vi "Periodic Tasks.vi"(8 "error in":errorcluster) -> ()   [LabVIEW 2017]
doc: "This VI runs in parallel to other tasks. It can contain as many user-defined periodic loops as you need. These can carry out PID or other sorts of timed response."
uses:
  <vilib>/Rock Robotics/WPI/Utilities/WPI_GetSetVariantRefNum.vi
  Robot Global Data.vi
  <vilib>/Rock Robotics/Network Tables/NT Write Numeric Array.vi
  <vilib>/Rock Robotics/Network Tables/NT Write Number.vi
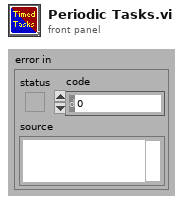
[diagram p1: front panel]
types:
  T1 = typedef "WPI_MotorControlDeviceRef.ctl" = cluster{"DeviceStatus":errorcluster, "Type":T2, "PWM":cluster{"PWM Channel":T3, "DeadBand":T4}, "CAN":cluster{"Device Number":u8, "SetOutput VI Ref":variant, "GetOutput VI Ref":variant, "Enable VI Ref":variant, "Disable VI Ref":variant, "Data":variant}, "Invert":bool, "DIO PWM":cluster{"PWM \"Enable\" Channel":T3, "DIOChannel":T5, "PWM Rate":dbl}}
  T2 = typedef "WPI_MotorControlType.ctl" = enum16{"PWM", "CAN", "DIO PWM"}
  T3 = typedef "FPGA_DIOPWMChannel.ctl" = enum8{"PWM 0", "PWM 1", "PWM 2", "PWM 3", "PWM 4", "PWM 5", "PWM 6", "PWM 7", "PWM 8", "PWM 9", "PWM MXP 0", "PWM MXP 1", "PWM MXP 2", "PWM MXP 3", "PWM MXP 4", "PWM MXP 5", "PWM MXP 6", "PWM MXP 7", "PWM MXP 8", "PWM MXP 9", "Invalid"}
  T4 = typedef "WPI_PWMDeadband.ctl" = cluster{"Name":string, "maxPositivePwm":i32, "minPositivePwm":i32, "centerPwm":i32, "maxNegativePwm":i32, "minNegativePwm":i32, "angularRange":u16}
  T5 = typedef "FPGA_DIOChannel.ctl" = enum8{"DIO 0", "DIO 1", "DIO 2", "DIO 3", "DIO 4", "DIO 5", "DIO 6", "DIO 7", "DIO 8", "DIO 9", "DIO MXP 0", "DIO MXP 1", "DIO MXP 2", "DIO MXP 3", "DIO MXP 4", "DIO MXP 5", "DIO MXP 6", "DIO MXP 7", "DIO MXP 8", "DIO MXP 9", "DIO MXP 10", "DIO MXP 11", "DIO MXP 12", "DIO MXP 13", "DIO MXP 14", "DIO MXP 15", "SPI Port CS1", "SPI Port CS2", "SPI Port CS3", "SPI Port MISO", "SPI Port MOSI", "Invalid"}
  T6 = typedef "WPI_RobotDriveDevRef.ctl" = cluster{"DevStatus":errorcluster, "Motors[]":T1[], "Square Inputs":bool, "Max Output":dbl}
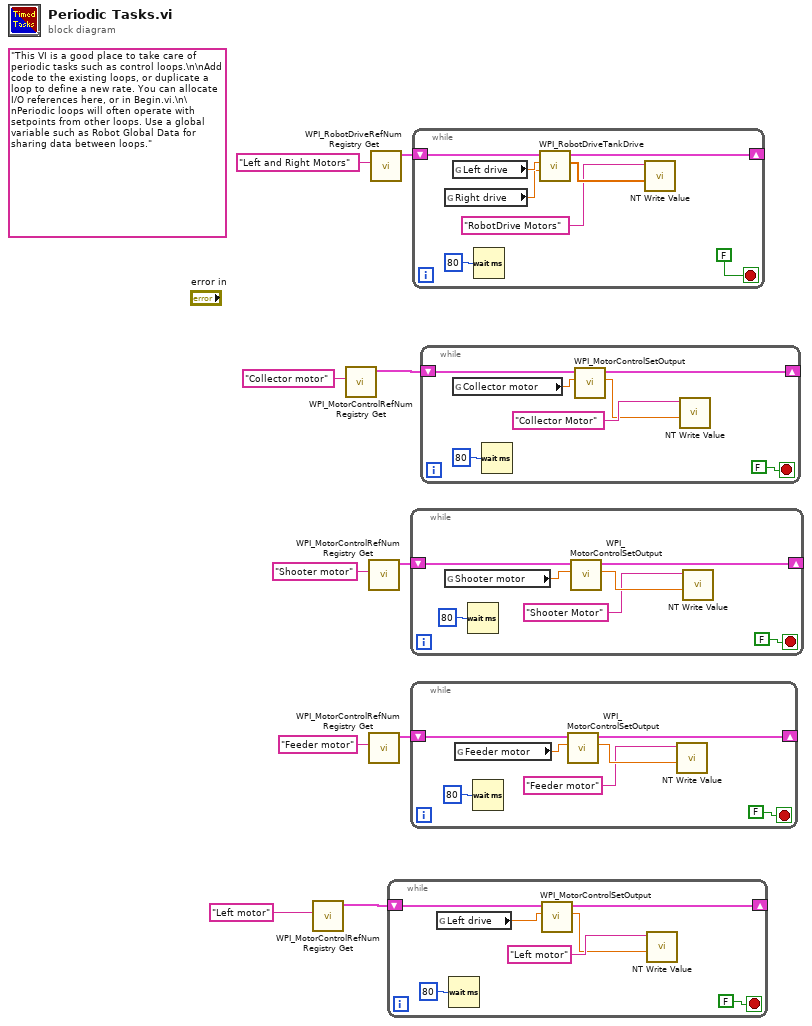
[diagram p0: block diagram]
diagram:
  (unwired) "This VI is a good place to take care of periodic tasks such as control loops.\n\nAdd code to the existing loops, or duplicate a loop to define a new rate. You can allocate I/O references here, or in Begin.vi.\n\nPeriodic loops will often operate with setpoints from other loops. Use a global variable such as Robot Global Data for sharing data between loops."
  n1 = call <vilib>:"WPI_MotorControlRefNum Registry Get.vi"("refnum name"="Left motor") -> ("MotorControlDevRef"=w2:T1)  [unwired: 9 in, 1 out]
  n2 = call <vilib>:"WPI_MotorControlRefNum Registry Get.vi"("refnum name"="Collector motor") -> ("MotorControlDevRef"=w5:T1)  [unwired: 9 in, 1 out]
  n3 = call <vilib>:"WPI_MotorControlRefNum Registry Get.vi"("refnum name"="Shooter motor") -> ("MotorControlDevRef"=w6:T1)  [unwired: 9 in, 1 out]
  n4 = call <vilib>:"WPI_MotorControlRefNum Registry Get.vi"("refnum name"="Feeder motor") -> ("MotorControlDevRef"=w3:T1)  [unwired: 9 in, 1 out]
  n5 = call <vilib>:"WPI_RobotDriveRefNum Registry Get.vi"("refnum name"="Left and Right Motors") -> ("RobotDriveDevRef"=w9:T6)  [unwired: 1 in, 9 out]
  n6 = while {
    shift-right: [w11] -> _
    shift-left: w2 -> [w12]
    stop <- FALSE stop-if-true
    n7 = global read "Robot Global Data.vi" "Left drive"() -> (w13:dbl)
    n8 = Wait (ms)(milliseconds to wait=u32 80) -> ()  [unwired: 1 out]
    n9 = call <vilib>:"WPI_MotorControlSetOutput.vi"("Output"=w13, "MotorControlDevRef"=w12) -> ("Motor Output"=w14:dbl, "MotorControlDevRef"=w11:T1)  [unwired: 7 in, 1 out]
    n10 = call-poly <vilib>:"NT Write Value.vi"("Numeric"=w14, "Name"="Left motor") -> ()  [unwired: 9 in, 1 out]
  }
  n11 = while {
    shift-right: [w20] -> _
    shift-left: w6 -> [w19]
    stop <- FALSE stop-if-true
    n12 = global read "Robot Global Data.vi" "Shooter motor"() -> (w22:dbl)
    n13 = Wait (ms)(milliseconds to wait=u32 80) -> ()  [unwired: 1 out]
    n14 = call <vilib>:"WPI_MotorControlSetOutput.vi"("Output"=w22, "MotorControlDevRef"=w19) -> ("Motor Output"=w21:dbl, "MotorControlDevRef"=w20:T1)  [unwired: 7 in, 1 out]
    n15 = call-poly <vilib>:"NT Write Value.vi"("Numeric"=w21, "Name"="Shooter Motor") -> ()  [unwired: 9 in, 1 out]
  }
  n16 = while {
    shift-right: [w27] -> _
    shift-left: w3 -> [w26]
    stop <- FALSE stop-if-true
    n17 = global read "Robot Global Data.vi" "Feeder motor"() -> (w29:dbl)
    n18 = Wait (ms)(milliseconds to wait=u32 80) -> ()  [unwired: 1 out]
    n19 = call <vilib>:"WPI_MotorControlSetOutput.vi"("Output"=w29, "MotorControlDevRef"=w26) -> ("Motor Output"=w28:dbl, "MotorControlDevRef"=w27:T1)  [unwired: 7 in, 1 out]
    n20 = call-poly <vilib>:"NT Write Value.vi"("Numeric"=w28, "Name"="Feeder motor") -> ()  [unwired: 9 in, 1 out]
  }
  n21 = while {
    shift-right: [w34] -> _
    shift-left: w9 -> [w35]
    stop <- FALSE stop-if-true
    n22 = global read "Robot Global Data.vi" "Right drive"() -> (w32:dbl)
    n23 = global read "Robot Global Data.vi" "Left drive"() -> (w33:dbl)
    n24 = Wait (ms)(milliseconds to wait=u32 80) -> ()  [unwired: 1 out]
    n25 = call <vilib>:"WPI_RobotDriveTankDrive.vi"("Right axis value"=w32, "Left axis value"=w33, "RobotDriveDevRef"=w35) -> ("Motor Values"=w37:dbl[], "RobotDriveDevRef"=w34:T6)  [unwired: 6 in, 1 out]
    n26 = call-poly <vilib>:"NT Write Value.vi"("Numeric Array"=w37, "Name"="RobotDrive Motors") -> ()  [unwired: 9 in, 1 out]
  }
  n27 = while {
    shift-right: [w40] -> _
    shift-left: w5 -> [w41]
    stop <- FALSE stop-if-true
    n28 = global read "Robot Global Data.vi" "Collector motor"() -> (w42:dbl)
    n29 = Wait (ms)(milliseconds to wait=u32 80) -> ()  [unwired: 1 out]
    n30 = call <vilib>:"WPI_MotorControlSetOutput.vi"("Output"=w42, "MotorControlDevRef"=w41) -> ("Motor Output"=w43:dbl, "MotorControlDevRef"=w40:T1)  [unwired: 7 in, 1 out]
    n31 = call-poly <vilib>:"NT Write Value.vi"("Numeric"=w43, "Name"="Collector Motor") -> ()  [unwired: 9 in, 1 out]
  }
